vi "SDCP TMC Encode.vi"(2 "error in (no error)":errorcluster, 3 "SDCP TMC Param":T1) -> (0 "error out":errorcluster, 1 "Encoded frame":u8[](array[numeric]))   [LabVIEW 2020]
uses:
  Typedefs/SDCP TMC Param.ctl
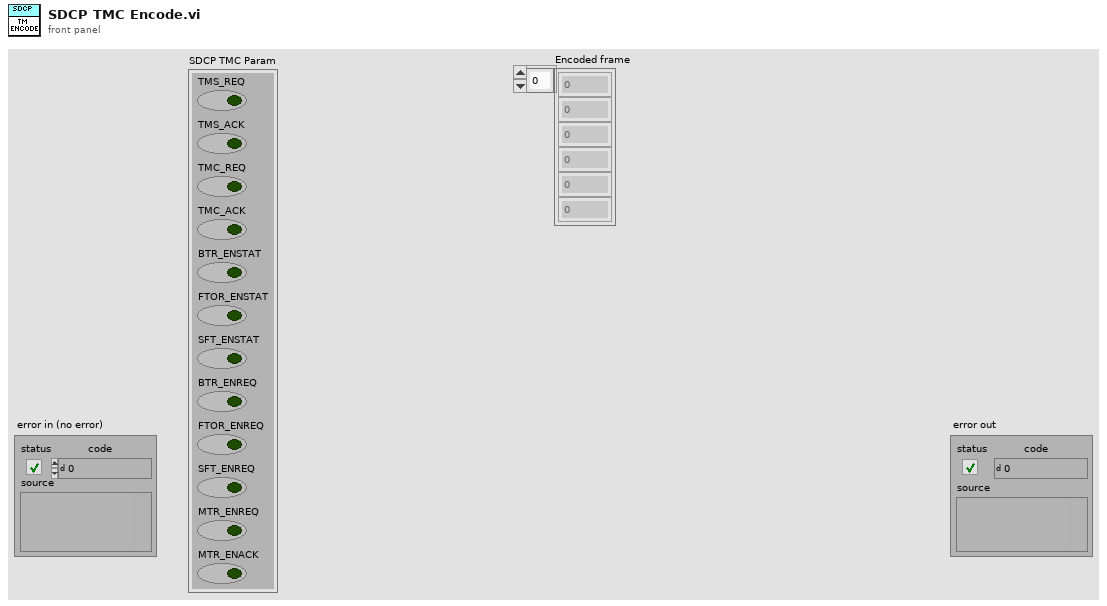
[diagram p1: front panel]
types:
  T1 = typedef "SDCP TMC Param.ctl" = cluster{"TMS_REQ":bool, "TMS_ACK":bool, "TMC_REQ":bool, "TMC_ACK":bool, "BTR_ENSTAT":bool, "FTOR_ENSTAT":bool, "SFT_ENSTAT":bool, "BTR_ENREQ":bool, "FTOR_ENREQ":bool, "SFT_ENREQ":bool, "MTR_ENREQ":bool, "MTR_ENACK":bool}
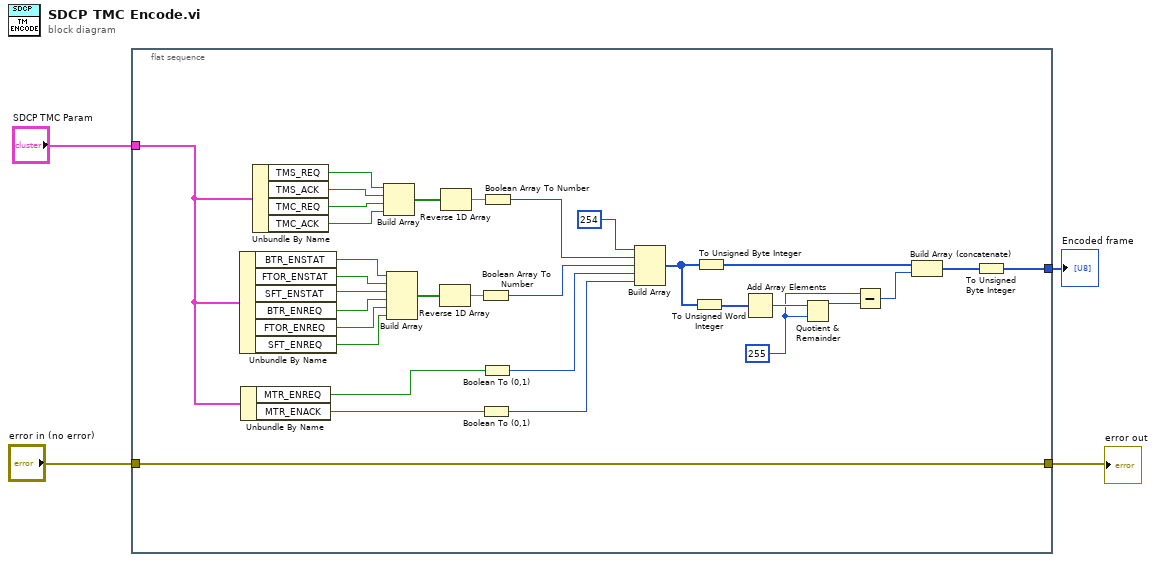
[diagram p0: block diagram]
diagram:
  n1 = flat-sequence {
    tunnel: "SDCP TMC Param" -> [w22]
    tunnel: "error in (no error)" -> [w7]
    tunnel: [w7] -> w2
    tunnel: [w5] -> w1
    frame #0 {
      w11 = u16 255 ("y")
      n2 = Unbundle By Name(w22) -> ("BTR_ENSTAT"=w30:bool, "FTOR_ENSTAT"=w29:bool, "SFT_ENSTAT"=w28:bool, "BTR_ENREQ"=w27:bool, "FTOR_ENREQ"=w26:bool, "SFT_ENREQ"=w25:bool)
      n3 = Unbundle By Name(w22) -> ("MTR_ENREQ"=w21:bool, "MTR_ENACK"=w20:bool)
      n4 = Unbundle By Name(w22) -> ("TMS_REQ"=w36:bool, "TMS_ACK"=w35:bool, "TMC_REQ"=w34:bool, "TMC_ACK"=w33:bool)
      n5 = Build Array(w36, w35, w34, w33) -> (w32:bool[])
      n6 = Build Array(w30, w29, w28, w27, w26, w25) -> (w24:bool[])
      n7 = Reverse 1D Array(array=w24) -> (reversed array=w23:bool[])
      n8 = Reverse 1D Array(array=w32) -> (reversed array=w31:bool[])
      n9 = Boolean Array To Number(Boolean array=w23) -> (number=w17:u32)
      n10 = Boolean To (0,1)(Boolean=w20) -> (0, 1=w15:i16)
      n11 = Boolean To (0,1)(Boolean=w21) -> (0, 1=w16:i16)
      n12 = Boolean Array To Number(Boolean array=w31) -> (number=w19:u32)
      n13 = Build Array(u32 254 ("element"), w19, w17, w16, w15) -> (w9:u32[])
      n14 = To Unsigned Word Integer(number=w9) -> (unsigned 16bit integer=w14:u16[])
      n15 = To Unsigned Byte Integer(number=w9) -> (unsigned 8bit integer=w8:u8[])
      n16 = Add Array Elements(numeric array=w14) -> (sum=w13:u16)
      n17 = Quotient & Remainder(x=w13, y=w11) -> (x-y*floor(x/y)=w12:u16)  [unwired: 1 out]
      n18 = Subtract(x=w11, y=w12) -> (x-y=w10:u16)
      n19 = Build Array (concatenate)(w8, w10) -> (w6:u16[])
      n20 = To Unsigned Byte Integer(number=w6) -> (unsigned 8bit integer=w5:u8[])
    }
  }
  "error out" <- w2
  "Encoded frame" <- w1
